vi "Initialize - Main Page Panel.vi"(8 "error in (no error)":errorcluster, 10 "Main Page References":T1, 11 "Item Ref in":T2 format="%.0x") -> (0 "error out":errorcluster, 3 "Item Ref out":T2 format="%.0x")   [LabVIEW 2019, in "UDP-Custom-Device System Explorer.lvlib"]
doc: "Initializes the Main Page front panel from the properties."
uses:
  UDP-Custom-Device System Explorer.lvlib
  <vilib>/NI VeriStand/Custom Device API/Custom Device Item Ref.ctl
  Types/Page References/Refs - Main Page.ctl
  <vilib>/NI VeriStand/Custom Device API/Custom Device API.lvlib
  Property Accessors/Main Accessors.lvlib
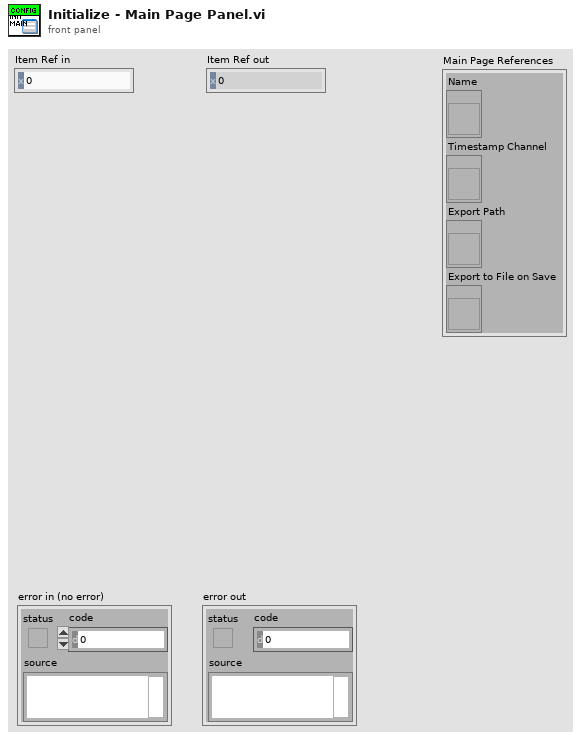
[diagram p1: front panel]
types:
  T1 = typedef "UDP-Custom-Device System Explorer.lvlib/Refs - Main Page.ctl" = cluster{"Name":refnum<vi>, "Timestamp Channel":refnum<vi>, "Export Path":refnum<vi>, "Export to File on Save":refnum<vi>}
  T2 = typedef "Custom Device API.lvlib/Custom Device Item Ref.ctl" = u64
  T3 = typedef "Custom Device API.lvlib/Custom Device Item Info.ctl" = cluster{"Name":string, "Is Channel":bool, "GUID":string, "Is Waveform":bool}
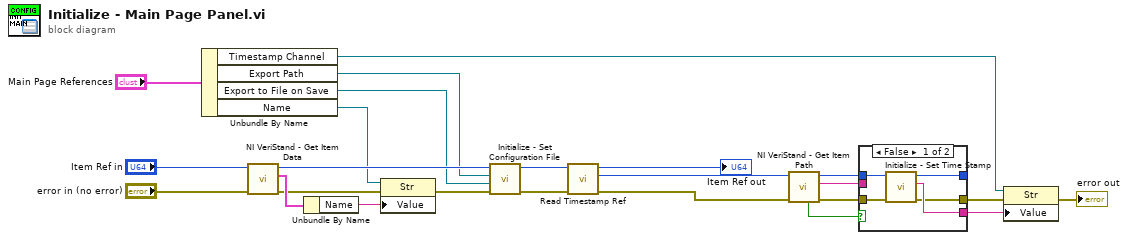
[diagram p0: block diagram]
diagram:
  n1 = Unbundle By Name("Main Page References") -> ("Timestamp Channel"=w6:refnum<vi>, "Export Path"=w9:refnum<vi>, "Export to File on Save"=w10:refnum<vi>, "Name"=w13:refnum<vi>)
  n2 = call <vilib>:"NI VeriStand - Get Item Data.vi"("error in (no error)"="error in (no error)", "Item Ref in"="Item Ref in") -> ("error out"=w12:errorcluster, "Item Info"=w15:T3, "Item Ref out"=w24:T2)  [unwired: 7 out]
  n3 = Unbundle By Name(w15) -> ("Name"=w16:string)
  n4 = property class="Str"(reference=w13, error in=w12, "Value"=w16) -> (error out=w11:errorcluster)  [unwired: 1 out]
  n5 = call "Initialize - Set Configuration File.vi"("error in (no error)"=w11, "Export to File on Save"=w10, "Export Path"=w9, "Item Ref in"=w24) -> ("error out"=w4:errorcluster, "Item Ref out"=w5:T2)  [unwired: 6 in]
  n6 = call "Read Timestamp Ref.vi"("error in (no error)"=w4, "Node Ptr"=w5) -> ("error out"=w2:errorcluster, "Timestamp Ref"=w1:T2, "Node Ptr out"=→"Item Ref out":T2)  [unwired: 7 in]
  n7 = call <vilib>:"NI VeriStand - Get Item Path.vi"("error in (no error)"=w2, "Item Ref in"=w1) -> ("error out"=w22:errorcluster, "Path"=w20:string, "Item Ref out"=w21:T2, "Found"=w19:bool)  [unwired: 6 in]
  n8 = case shown="False" w19 {
    tunnel: w20 -> [_ w31]
    tunnel: w21 -> [w28 w32]
    tunnel: w22 -> [w29 w30]
    tunnel: [w27 w32] -> _
    tunnel: [w26 w31] -> w23
    tunnel: [w25 w30] -> w8
    frame False {
      n9 = call "Initialize - Set Time Stamp.vi"("error in (no error)"=w29, "Device Item Ref in"=w28) -> ("error out"=w25:errorcluster, "Path"=w26:string, "Device Item Ref out"=w27:T2)  [unwired: 7 in]
    }
    frame True {
    }
  }
  n10 = property class="Str"(reference=w6, error in=w8, "Value"=w23) -> (error out=→"error out":errorcluster)  [unwired: 1 out]
